vi "get lengths.vi"(8 "error in":errorcluster, 9 "Timeout (ms)":i32=-1, 11 "profibus reference":T2) -> (0 "error out":errorcluster, 2 "Slave Info List":T1(array[cluster]), 3 "profibus reference out":T2)   [LabVIEW 2013, in "dynamic profibus.lvlib"]
uses:
  dynamic profibus.lvlib
  fpga reference.ctl
  profibus master action.ctl
  <vilib>/rvi/interface/common/niFpgaWaitOnOcc.vi
  <vilib>/Utility/error.llb/Error Cluster From Error Code.vi
  <vilib>/rvi/errors/niLvFpgaAdjustHostInterfaceError.vi
  <vilib>/rvi/interface/nirviMethod/nirviMethod.xnode
  <vilib>/rvi/errors/niLvFpgaMergeErrorWithErrorCode.vi
  <vilib>/NI/Configuration Framework/NISE_CEF_TreeControl.lvlib
  <vilib>/FPGAPlugInAG/Dynamic/niLvFpga_WriteFifo_Dynamic.vi
  <vilib>/FPGAPlugInAG/Dynamic/niLvFpga_ReadFifo_Dynamic.vi
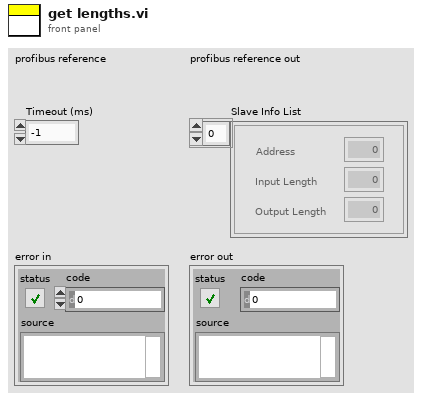
[diagram p1: front panel]
types:
  T1 = cluster{"Address":i8, "Input Length":u8, "Output Length":u8}[]
  T2 = typedef "dynamic profibus.lvlib/fpga reference.ctl" = refnum<k20>
  T3 = typedef "dynamic profibus.lvlib/profibus master action.ctl" = enum8{"initialize", "uninitialize", "stop", "get input", "get input size", "set output", "get output size", "get diagnostic", "transfer data", "transfer diagnostics"}
  T4 = cluster{"Address":i8, "Input Length":u8, "Output Length":u8}
  T5 = typedef "dynamic profibus.lvlib/profibus master transmit header.ctl" = enum8{"Error", "Input", "Diagnostic", "input size", "output size"}
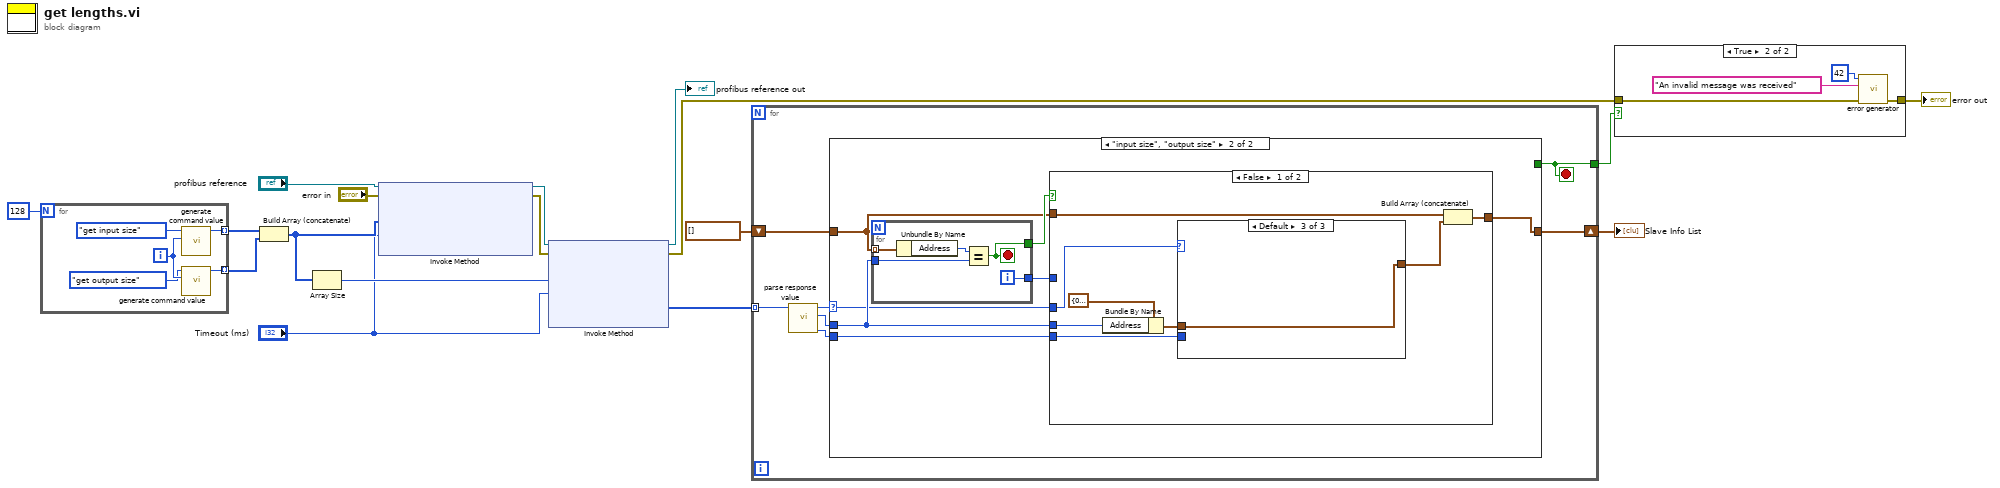
[diagram p0: block diagram]
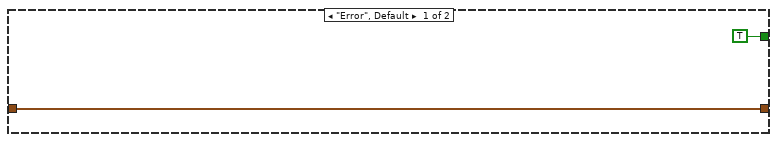
[diagram p3: hidden frame]
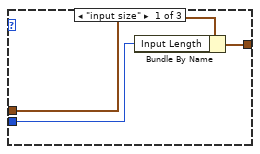
[diagram p4: hidden frame]
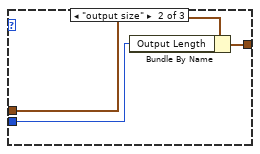
[diagram p5: hidden frame]
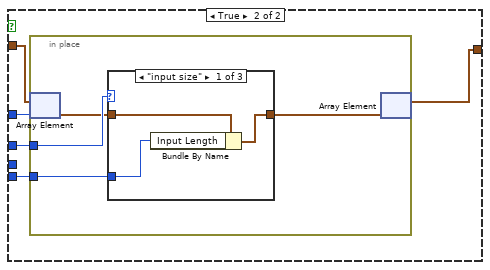
[diagram p6: hidden frame]
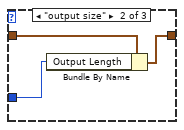
[diagram p7: hidden frame]
diagram:
  n1 = for {
    N: 128 -> [_]
    tunnel: [w19] -> w13 mode=indexing
    tunnel: [w18] -> w12 mode=indexing
    i -> [w21]
    n2 = call "generate command value.vi"("device"=w21, "action"=profibus_master_action."get input size") -> ("Element"=w18:u32)  [unwired: 9 in]
    n3 = call "generate command value.vi"("device"=w21, "action"=profibus_master_action."get output size") -> ("Element"=w19:u32)  [unwired: 9 in]
  }
  n4 = Build Array (concatenate)(w12, w13) -> (w9:u32[])
  n5 = Array Size(array=w9) -> (size(s)=w8:i32)
  n6 = xnode "Invoke Method"("FPGA VI Reference In"="profibus reference", "error in"="error in", "Data"=w9, "Timeout (ms)"="Timeout (ms)") -> ("FPGA VI Reference Out"=w11:T2, "error out"=w16:errorcluster)  [unwired: 1 out]
  n7 = xnode "Invoke Method"("FPGA VI Reference In"=w11, "error in"=w16, "Number of Elements"=w8, "Timeout (ms)"="Timeout (ms)") -> ("FPGA VI Reference Out"=→"profibus reference out":T2, "error out"=w2:errorcluster, "Data"=w6:u32[])  [unwired: 1 out]
  n8 = for {
    tunnel: w6 -> [w29] mode=indexing
    shift-right: [w24] -> w4
    shift-left: T1 [] ("Slave Info List") -> [w25]
    tunnel: [w23] -> w3
    stop <- w23 stop-if-true
    n9 = call "parse response value.vi"("Element"=w29) -> ("data"=w26:u8, "device"=w27:u8, "header"=w28:T5)  [unwired: 7 in, 1 out]
    n10 = case shown="\"input size\", \"output size\"" w28 {
      selector: w28 -> [_ w32]
      tunnel: w27 -> [_ w34]
      tunnel: w26 -> [_ w33]
      tunnel: w25 -> [w31 w36]
      tunnel: [w31 w35] -> w24
      tunnel: [TRUE _] -> w23
      frame "Error", Default {
      }
      frame "input size", "output size" {
        n11 = for {
          tunnel: w36 -> [w74] mode=indexing
          tunnel: w34 -> [w72]
          tunnel: [w70] -> w38
          tunnel: [w71] -> w37
          i -> [w71]
          stop <- w70 stop-if-true
          n12 = Unbundle By Name(w74) -> ("Address"=w73:i8)
          n13 = Equal?(x=w73, y=w72) -> (x = y?=w70:bool)
        }
        n14 = case shown="False" w38 {
          tunnel: w37 -> [_ w58]
          tunnel: w36 -> [w46 w57]
          tunnel: [w45 w56] -> w35
          tunnel: w34 -> [w43 _]
          tunnel: w33 -> [w39 w54]
          tunnel: w32 -> [w42 w55]
          frame False {
            n15 = Bundle By Name(cluster=T4 {"Address"=0, "Input Length"=0, "Output Length"=0} ("Slave Info"), "Address"=w43) -> (w41:T4)
            n16 = case shown="Default" w42 {
              tunnel: w41 -> [w49 w52 w53]
              tunnel: [w48 w51 w53] -> w40
              tunnel: w39 -> [w47 w50 _]
              frame "input size" {
                n17 = Bundle By Name(cluster=w49, "Input Length"=w47) -> (w48:T4)
              }
              frame "output size" {
                n18 = Bundle By Name(cluster=w52, "Output Length"=w50) -> (w51:T4)
              }
              frame Default {
              }
            }
            n19 = Build Array (concatenate)(w46, w40) -> (w45:T1)
          }
          frame True {
            n20 = in-place {
              in-place-border: w55 -> [w62]
              in-place-border: w54 -> [w59]
              n21 = in-place-array #1(w57, w58) -> (w61:T4)
              n22 = case shown="\"input size\"" w62 {
                tunnel: w61 -> [w65 w68 w69]
                tunnel: [w64 w67 w69] -> w60
                tunnel: w59 -> [w63 w66 _]
                frame "input size" {
                  n23 = Bundle By Name(cluster=w65, "Input Length"=w63) -> (w64:T4)
                }
                frame "output size" {
                  n24 = Bundle By Name(cluster=w68, "Output Length"=w66) -> (w67:T4)
                }
                frame Default {
                }
              }
              n25 = in-place-array #1(w60) -> (w56:T1)  [unwired: 1 out]
            }
          }
        }
      }
    }
  }
  "Slave Info List" <- w4
  n26 = case shown="True" w3 {
    tunnel: w2 -> [w75 w79]
    tunnel: [w75 w78] -> w1
    frame False {
    }
    frame True {
      n27 = call <vilib>:"error generator.vi"("error in"=w79, "append error message"="An invalid message was received", "error code (0)"=42) -> ("error out"=w78:errorcluster)  [unwired: 6 in]
    }
  }
  "error out" <- w1
